vi "Fetch Idle Pattern Frame.vi"(10 "Effect":T1) -> (2 "Array":u16[](array[numeric]))   [LabVIEW 2026]
uses:
  Idle Pattern.ctl
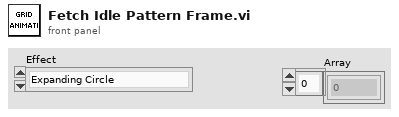
[diagram p1: front panel]
types:
  T1 = typedef "Idle Pattern.ctl" = enum16{"Expanding Circle", "Plasma", "Radar Sweep", "Matrix Rain", "Campfire", "Diagonal Scan", "LV40"}
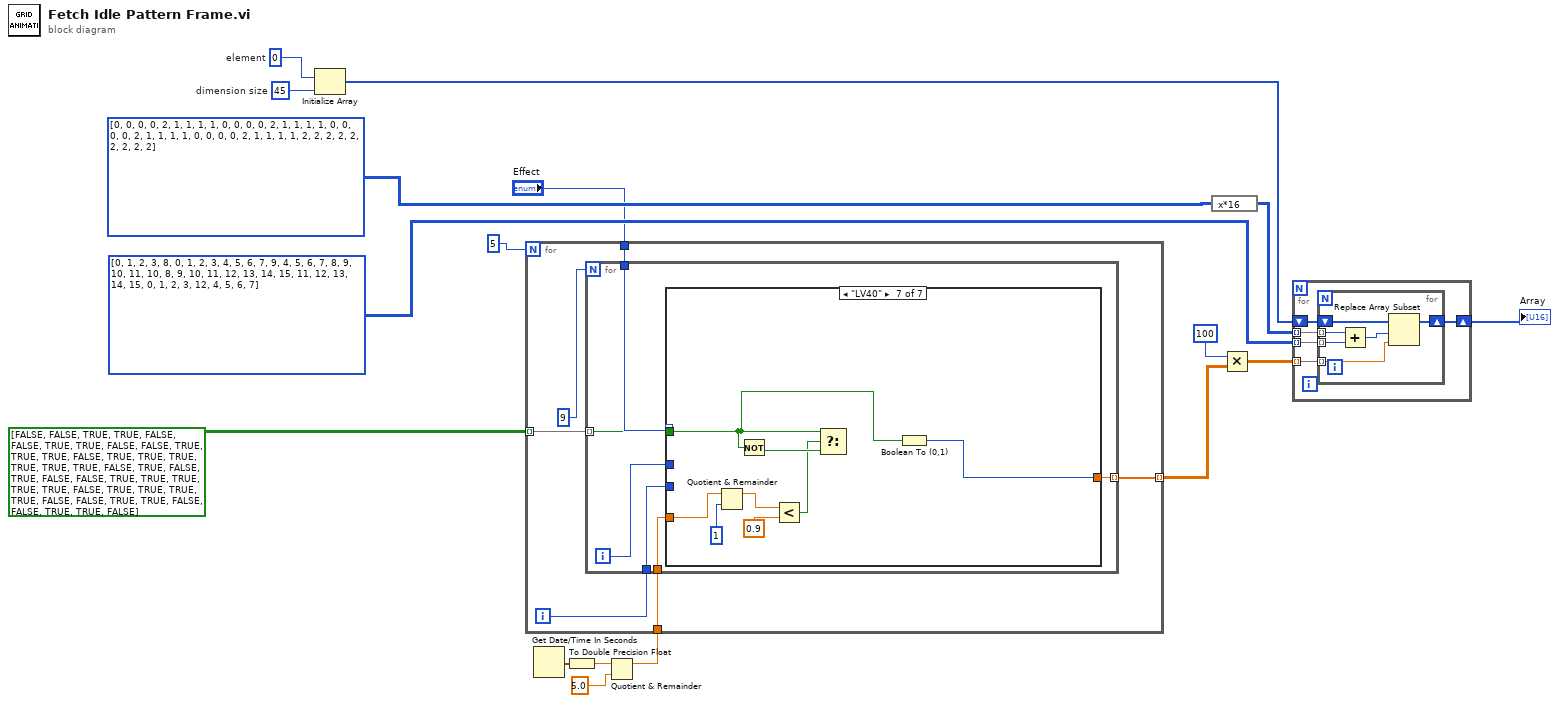
[diagram p0: block diagram]
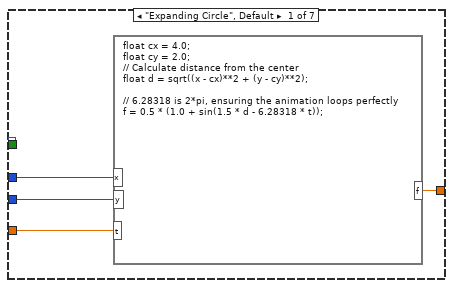
[diagram p2: hidden frame]
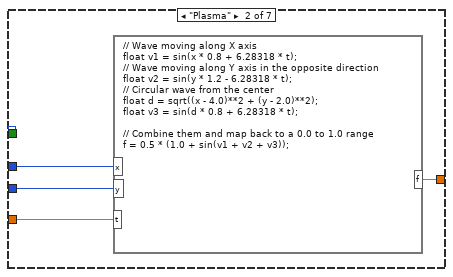
[diagram p3: hidden frame]
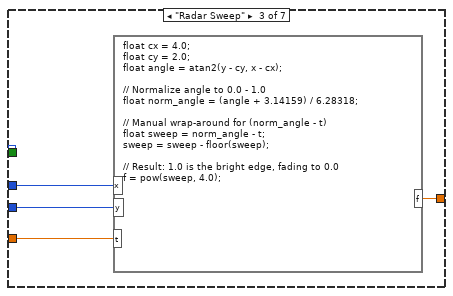
[diagram p4: hidden frame]
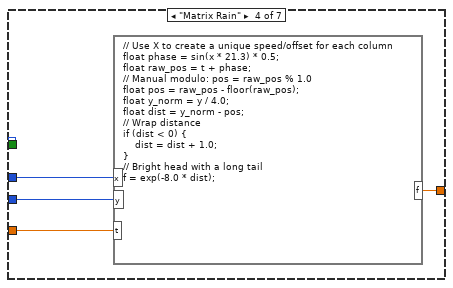
[diagram p5: hidden frame]
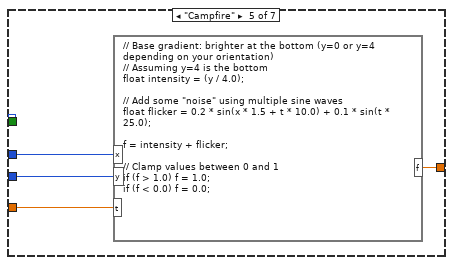
[diagram p6: hidden frame]
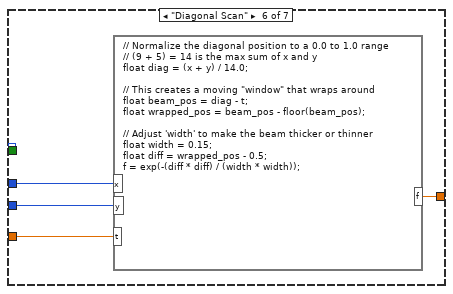
[diagram p7: hidden frame]
diagram:
  w16 = u16 0  # element
  w17 = 45  # dimension size
  n1 = Initialize Array(w16, w17) -> (w15:u16[])
  n2 = Get Date/Time In Seconds() -> (seconds since 1Jan1904=w11:timestamp)
  n3 = To Double Precision Float(number=w11) -> (double precision float=w10:dbl)
  n4 = Quotient & Remainder(x=w10, y=5.0) -> (x-y*floor(x/y)=w8:dbl)  [unwired: 1 out]
  n5 = for {
    N: 5 -> [_]
    tunnel: w8 -> [w21]
    tunnel: [w20] -> w6 mode=indexing
    tunnel: "Effect" -> [w19]
    tunnel: bool[][] [[FALSE, FALSE, TRUE, TRUE, FALSE, FALSE, TRUE, TRUE, FALSE], [FALSE, TRUE, TRUE, TRUE, FALSE, TRUE, TRUE, TRUE, TRUE], [TRUE, TRUE, FALSE, TRUE, FALSE, TRUE, FALSE, FALSE, TRUE], [TRUE, TRUE, TRUE, TRUE, FALSE, TRUE, TRUE, TRUE, TRUE], [FALSE, FALSE, TRUE, TRUE, FALSE, FALSE, TRUE, TRUE, FALSE]] -> [w18] mode=indexing
    i -> [w22]
    n6 = for {
      N: 9 -> [_]
      tunnel: w22 -> [w28]
      tunnel: w21 -> [w27]
      tunnel: [w26] -> w20 mode=indexing
      tunnel: w19 -> [w25]
      tunnel: w18 -> [w24] mode=indexing
      i -> [w29]
      n7 = case shown="\"LV40\"" w25 {
        tunnel: w29 -> [w33 w37 w41 w45 w49 w53 _]
        tunnel: w28 -> [w32 w36 w40 w44 w48 w52 _]
        tunnel: w27 -> [w31 w35 w39 w43 w47 w51 w57]
        tunnel: [w30 w34 w38 w42 w46 w50 w60] -> w26
        tunnel: w24 -> [_ _ _ _ _ _ w58]
        frame "Expanding Circle", Default {
          n8 = formula code="float cx = 4.0;\nfloat cy = 2.0;\n// Calculate distance from the center\nfloat d = sqrt((x - cx)**2 + (y - cy)**2);\n\n// 6.28318 is 2*pi, ensuring the animation loops perfectly\nf = 0.5 * (1.0 + sin(1.5 * d - 6.28318 * t));"("x"=w33, "y"=w32, "t"=w31) -> ("f"=w30:dbl)
        }
        frame "Plasma" {
          n9 = formula code="// Wave moving along X axis\nfloat v1 = sin(x * 0.8 + 6.28318 * t);\n// Wave moving along Y axis in the opposite direction\nfloat v2 = sin(y * 1.2 - 6.28318 * t);\n// Circular wave from the center\nfloat d = sqrt((x - 4.0)**2 + (y - 2.0)**2);\nfloat v3 = sin(d * 0.8 + 6.28318 * t);\n\n// Combine them and map back to a 0.0 to 1.0 range\nf = 0.5 * (1.0 + sin(v1 + v2 + v3));"("x"=w37, "y"=w36, "t"=w35) -> ("f"=w34:dbl)
        }
        frame "Radar Sweep" {
          n10 = formula code="float cx = 4.0;\nfloat cy = 2.0;\nfloat angle = atan2(y - cy, x - cx);\n\n// Normalize angle to 0.0 - 1.0\nfloat norm_angle = (angle + 3.14159) / 6.28318;\n\n// Manual wrap-around for (norm_angle - t)\nfloat sweep = norm_angle - t;\nsweep = sweep - floor(sweep); \n\n// Result: 1.0 is the bright edge, fading to 0.0\nf = pow(sweep, 4.0);"("x"=w41, "y"=w40, "t"=w39) -> ("f"=w38:dbl)
        }
        frame "Matrix Rain" {
          n11 = formula code="// Use X to create a unique speed/offset for each column\nfloat phase = sin(x * 21.3) * 0.5; \nfloat raw_pos = t + phase;\n// Manual modulo: pos = raw_pos % 1.0\nfloat pos = raw_pos - floor(raw_pos);\nfloat y_norm = y / 4.0;\nfloat dist = y_norm - pos;\n// Wrap distance\nif (dist < 0) {\n    dist = dist + 1.0;\n}\n// Bright head with a long tail\nf = exp(-8.0 * dist);"("x"=w45, "y"=w44, "t"=w43) -> ("f"=w42:dbl)
        }
        frame "Campfire" {
          n12 = formula code="// Base gradient: brighter at the bottom (y=0 or y=4 depending on your orientation)\n// Assuming y=4 is the bottom\nfloat intensity = (y / 4.0);\n\n// Add some \"noise\" using multiple sine waves\nfloat flicker = 0.2 * sin(x * 1.5 + t * 10.0) + 0.1 * sin(t * 25.0);\n\nf = intensity + flicker;\n\n// Clamp values between 0 and 1\nif (f > 1.0) f = 1.0;\nif (f < 0.0) f = 0.0;"("x"=w49, "y"=w48, "t"=w47) -> ("f"=w46:dbl)
        }
        frame "Diagonal Scan" {
          n13 = formula code="// Normalize the diagonal position to a 0.0 to 1.0 range\n// (9 + 5) = 14 is the max sum of x and y\nfloat diag = (x + y) / 14.0; \n\n// This creates a moving \"window\" that wraps around\nfloat beam_pos = diag - t;\nfloat wrapped_pos = beam_pos - floor(beam_pos);\n\n// Adjust 'width' to make the beam thicker or thinner\nfloat width = 0.15;\nfloat diff = wrapped_pos - 0.5;\nf = exp(-(diff * diff) / (width * width));"("x"=w53, "y"=w52, "t"=w51) -> ("f"=w50:dbl)
        }
        frame "LV40" {
          n14 = Quotient & Remainder(x=w57, y=1) -> (x-y*floor(x/y)=w56:dbl)  [unwired: 1 out]
          n15 = Not(x=w58) -> (.not. x?=w59:bool)
          n16 = Less?(x=w56, y=0.9) -> (x < y?=w54:bool)
          n17 = Select(t=w58, s=w54, f=w59) -> ()  [unwired: 1 out]
          n18 = Boolean To (0,1)(Boolean=w58) -> (0, 1=w60:i16)
        }
      }
    }
  }
  n19 = expression code="x*16"(i32[][] [[0, 0, 0, 0, 2, 1, 1, 1, 1], [0, 0, 0, 0, 2, 1, 1, 1, 1], [0, 0, 0, 0, 2, 1, 1, 1, 1], [0, 0, 0, 0, 2, 1, 1, 1, 1], [2, 2, 2, 2, 2, 2, 2, 2, 2]]) -> (w3:i32[][])
  n20 = Multiply(x=100, y=w6) -> (x*y=w5:dbl[][])
  n21 = for {
    shift-right: [w65] -> w2
    shift-left: w15 -> [w66]
    tunnel: w5 -> [w64] mode=indexing
    tunnel: w3 -> [w63] mode=indexing
    tunnel: i32[][] [[0, 1, 2, 3, 8, 0, 1, 2, 3], [4, 5, 6, 7, 9, 4, 5, 6, 7], [8, 9, 10, 11, 10, 8, 9, 10, 11], [12, 13, 14, 15, 11, 12, 13, 14, 15], [0, 1, 2, 3, 12, 4, 5, 6, 7]] -> [w62] mode=indexing
    n22 = for {
      shift-right: [w71] -> w65
      shift-left: w66 -> [w72]
      tunnel: w64 -> [w70] mode=indexing
      tunnel: w63 -> [w69] mode=indexing
      tunnel: w62 -> [w68] mode=indexing
      n23 = Add(x=w69, y=w68) -> (x+y=w67:i32)
      n24 = Replace Array Subset(array=w72, new element=w70, index=w67) -> (w71:u16[])
    }
  }
  "Array" <- w2
